vi "StartCommand.vi"(1 "Control":T1) -> (0 "String":string)   [LabVIEW 2023]
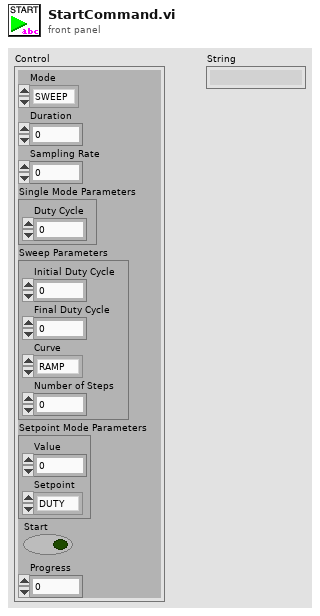
[diagram p1: front panel]
types:
  T1 = cluster{"Mode":enum16{"SWEEP", "SETPOINT", "SINGLE"}, "Duration":dbl, "Sampling Rate":dbl, "Single Mode Parameters":cluster{"Duty Cycle":u8}, "Sweep Parameters ":cluster{"Initial Duty Cycle":u8, "Final Duty Cycle":u8, "Curve":enum16{"RAMP", "STEPS"}, "Number of Steps":u8}, "Setpoint Mode Parameters":cluster{"Value":dbl, "Setpoint":enum16{"DUTY", "RPM", "POWER", "THRUST"}}, "Start":bool, "Progress":u8}
  T2 = cluster{"Initial Duty Cycle":u8, "Final Duty Cycle":u8, "Curve":enum16{"RAMP", "STEPS"}, "Number of Steps":u8}
  T3 = cluster{"Value":dbl, "Setpoint":enum16{"DUTY", "RPM", "POWER", "THRUST"}}
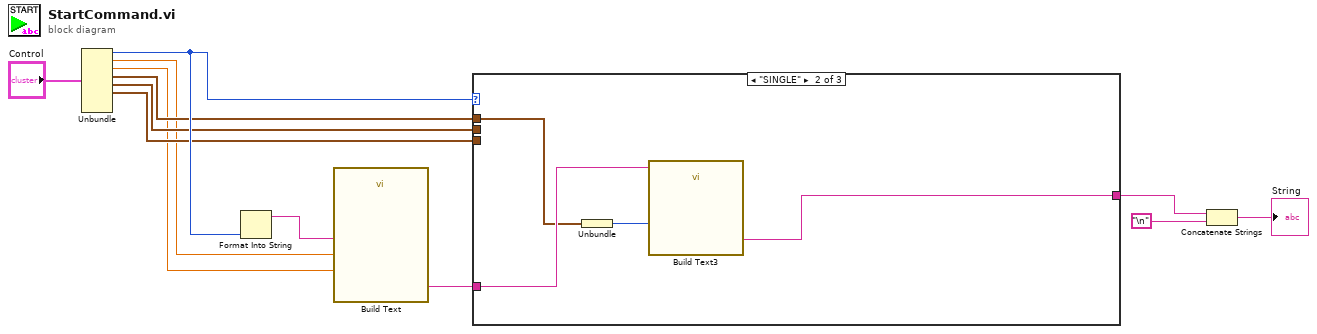
[diagram p0: block diagram]
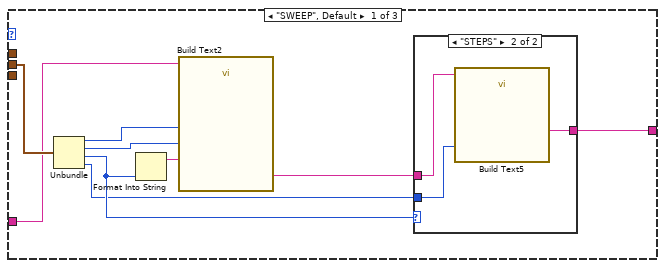
[diagram p2: hidden frame]
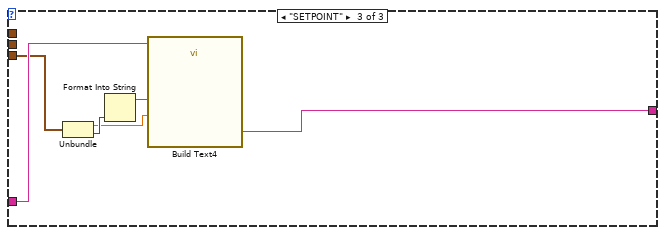
[diagram p4: hidden frame]
diagram:
  n1 = Unbundle("Control") -> ("Mode"=w12:enum16{"SWEEP", "SETPOINT", "SINGLE"}, "Duration"=w2:dbl, "Sampling Rate"=w3:dbl, "Single Mode Parameters"=w5:cluster{"Duty Cycle":u8}, "Sweep Parameters"=w11:T2, "Setpoint Mode Parameters"=w6:T3)  [unwired: 2 out]
  n2 = Format Into String(w12) -> (resulting string=w1:string)  [unwired: 3 in, 1 out]
  n3 = call "Build Text"("MODE"=w1, "DURATION"=w2, "SAMPLING_RATE"=w3) -> ("Result"=w4:string)  [unwired: 11 in, 1 out]
  n4 = case shown="\"SINGLE\"" w12 {
    tunnel: w4 -> [w17 w29 w35]
    tunnel: w5 -> [_ w28 _]
    tunnel: w11 -> [w21 _ _]
    tunnel: w6 -> [_ _ w34]
    tunnel: [w15 w26 w30] -> w8
    frame "SWEEP", Default {
      n5 = Unbundle(w21) -> ("Initial Duty Cycle"=w20:u8, "Final Duty Cycle"=w19:u8, "Curve"=w16:enum16{"RAMP", "STEPS"}, "Number of Steps"=w13:u8)
      n6 = Format Into String(w16) -> (resulting string=w18:string)  [unwired: 3 in, 1 out]
      n7 = call "Build Text2"("Beginning Text"=w17, "INITIAL_DC"=w20, "FINAL_DC"=w19, "CURVE"=w18) -> ("Result"=w14:string)  [unwired: 10 in, 1 out]
      n8 = case shown="\"STEPS\"" w16 {
        tunnel: [w22 w24] -> w15
        tunnel: w14 -> [w22 w25]
        tunnel: w13 -> [_ w23]
        frame "RAMP", Default {
        }
        frame "STEPS" {
          n9 = call "Build Text5"("Beginning Text"=w25, "N_STEPS"=w23) -> ("Result"=w24:string)  [unwired: 12 in, 1 out]
        }
      }
    }
    frame "SINGLE" {
      n10 = Unbundle(w28) -> ("Duty Cycle"=w27:u8)
      n11 = call "Build Text3"("Beginning Text"=w29, "DUTY_CYCLE"=w27) -> ("Result"=w26:string)  [unwired: 12 in, 1 out]
    }
    frame "SETPOINT" {
      n12 = Unbundle(w34) -> ("Value"=w31:dbl, "Setpoint"=w33:enum16{"DUTY", "RPM", "POWER", "THRUST"})
      n13 = Format Into String(w33) -> (resulting string=w32:string)  [unwired: 3 in, 1 out]
      n14 = call "Build Text4"("Beginning Text"=w35, "SETPOINT"=w32, "VALUE"=w31) -> ("Result"=w30:string)  [unwired: 11 in, 1 out]
    }
  }
  n15 = Concatenate Strings(w8, "\n") -> (→"String":string)
